vi "Run.vi"(7 "Data":refnum<class "Datum.lvclass">, 8 "Error In":errorcluster, 11 "Compiler In":refnum<class "Compiler.lvclass">) -> (0 "Error Out":errorcluster, 3 "Compiler Out":refnum<class "Compiler.lvclass">)   [LabVIEW 2018, in "Toolkit.lvlib" / "Compiler.lvclass"]
uses:
  Compiler.lvclass
  Data/Datum/Datum.lvclass
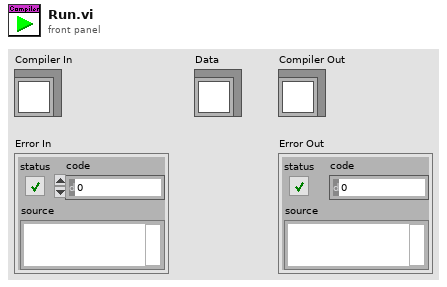
[diagram p1: front panel]
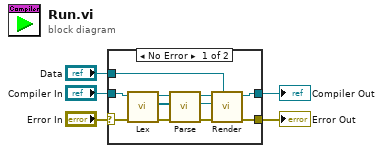
[diagram p0: block diagram]
diagram:
  n1 = case shown="No Error" "Error In" {
    selector: "Error In" -> [w8 w17]
    tunnel: "Compiler In" -> [w9 w18]
    tunnel: [w7 w18] -> w3
    tunnel: [w6 w17] -> w2
    tunnel: "Data" -> [w10 _]
    frame No Error {
      n2 = call-dynamic "Lex.vi"("Error In"=w8, "Compiler In"=w9) -> ("Error Out"=w15:errorcluster, "Tokens"=w14:refnum<class "Token.lvclass">[], "Compiler Out"=w16:refnum<class "Compiler.lvclass">)  [unwired: 7 in]
      n3 = call-dynamic "Parse.vi"("Error In"=w15, "Tokens"=w14, "Compiler In"=w16) -> ("Error Out"=w11:errorcluster, "Abstract Syntax Tree"=w12:refnum<class "Root.lvclass">, "Compiler Out"=w13:refnum<class "Compiler.lvclass">)  [unwired: 6 in]
      n4 = call "Render.vi"("Data"=w10, "Error In"=w11, "Abstract Syntax Tree"=w12, "Compiler In"=w13) -> ("Error Out"=w6:errorcluster, "Compiler Out"=w7:refnum<class "Compiler.lvclass">)  [unwired: 6 in]
    }
    frame Error {
    }
  }
  "Compiler Out" <- w3
  "Error Out" <- w2
